vi "Client Console.vi"() -> ()   [LabVIEW 2020]
uses:
  _addons/TCP-Router/_support/tcp-msg type.ctl
  <vilib>/event_ctls.llb/eventvkey.ctl
  <vilib>/Utility/High Resolution Relative Seconds.vi
  <userlib>/_NEVSTOP/Communicable State Machine(CSM)/AdvanceAPI/CSM - Keywords.vi
  <userlib>/_NEVSTOP/Communicable State Machine(CSM)/_Shared/Trim Single-line Text.vi
  <userlib>/_NEVSTOP/Communicable State Machine(CSM)/addons/API-String-Arugments-Support/API String Arguments Support.lvlib
  <userlib>/_NEVSTOP/Communicable State Machine(CSM)/Communicable State Machine.lvlib
  <userlib>/_NEVSTOP/Communicable State Machine(CSM)/addons/INI-Static-Variable-Support/INI-Static-Variable-Support.lvlib
  _addons/TCP-Router/CSM-TCP-Router.lvlib
  <userlib>/_NEVSTOP/Communicable State Machine(CSM)/_Shared/CSM Shared.lvlib
panel:
  out "History Length(Char)":i32
  out "TCP LoopTime(s)":dbl format="%#_3g"
  out "Queue LoopTime(s)":dbl format="%#_3g"
  out "#Queue Backog":i32
  in  "Exit":bool
  out "Console":string
  in  "Command":string caption="$"
  out "To Who":string
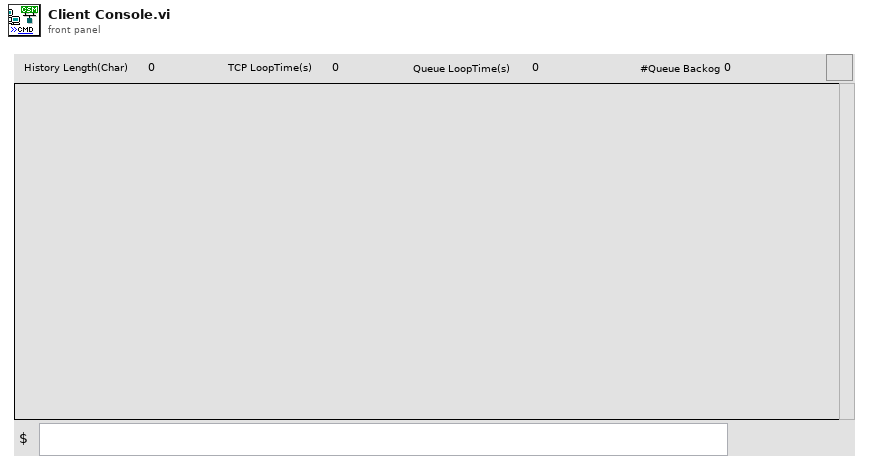
[diagram p1: front panel]
types:
  T1 = typedef "CSM-TCP-Router.lvlib/tcp-msg type.ctl" = enum8{"info", "error", "cmd", "cmd-resp", "resp", "async-resp", "status", "interrupt"}
  T2 = typedef "eventvkey.ctl" = enum16{"ASCII", "Enter", "Return", "Shift", "Ctrl", "Alt", "Cmd", "Opt", "Caps", "NumLock", "Clear", "Break", "Up", "Down", "Left", "Right", "Insert", "Delete", "Home", "End", "PageUp", "PageDown", "Escape", "Help", "Pause", "ScrollLock", "F1", "F2", "F3", "F4", "F5", "F6", "F7", "F8", "F9", "F10", "F11", "F12", "F13", "F14", "F15", "F16", "F17", "F18", "F19", "F20", "F21", "F22", "F23", "F24", "Play", "VolumeUp", "VolumeDown", "Mute", "Two Byte Char"}
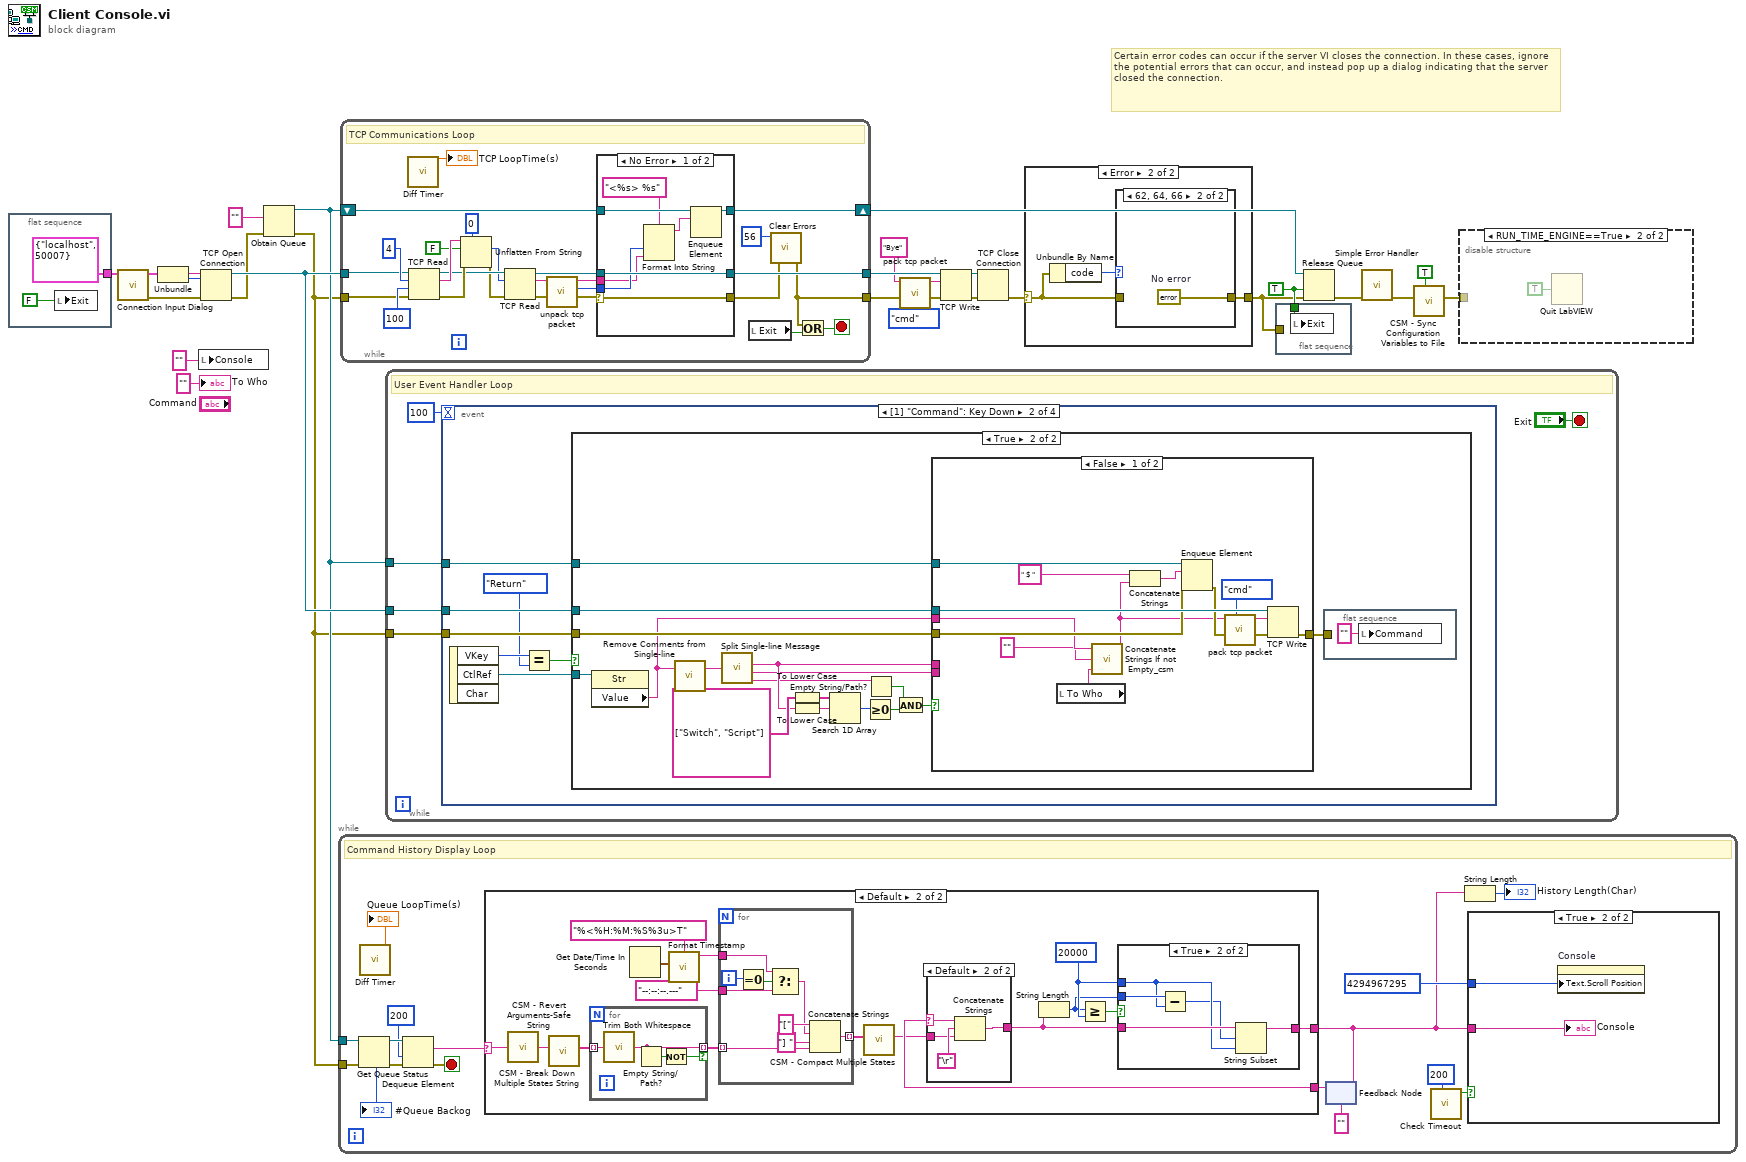
[diagram p0: block diagram]
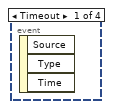
[diagram p7: hidden frame]
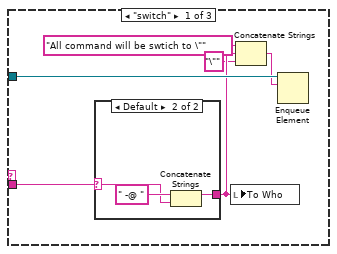
[diagram p10: hidden frame]
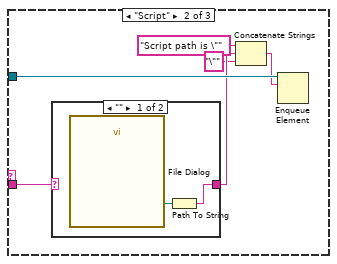
[diagram p12: hidden frame]
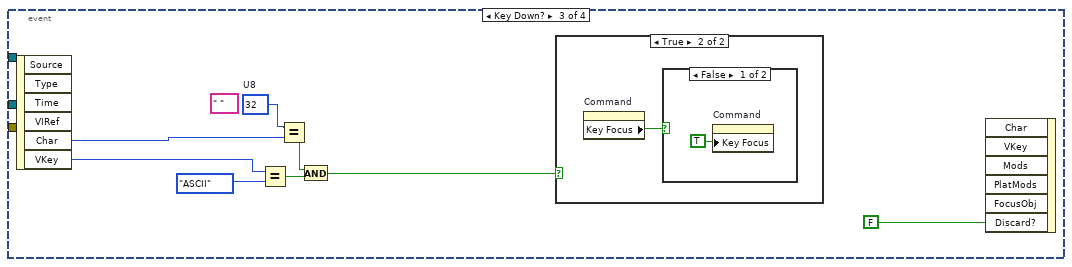
[diagram p14: hidden frame]
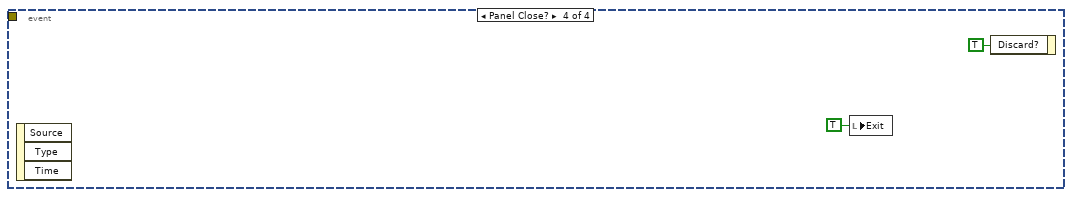
[diagram p17: hidden frame]
diagram:
  w6 = TRUE ("force destroy? (F)")
  # "Certain error codes can occur if the server VI closes the connection. In these cases, ignore the potential errors that can occur, and instead pop up a dialog indicating that the server closed the connection."
  n1 = flat-sequence {
    tunnel: [cluster{"IP Address":string, "Port":u16} {"IP Address"="localhost", "Port"=50007} ("Connection Info")] -> w16
    frame #0 {
      n2 = local write "Exit"(FALSE ("exit")) -> ()
    }
  }
  n3 = call "Connection Input Dialog.vi"("Connection Info"=w16) -> ("Error out"=w15:errorcluster, "Connection Info output"=w14:cluster{"IP Address":string, "Port":u16})  [unwired: 9 in]
  n4 = Unbundle(w14) -> ("IP Address"=w13:string, "Port"=w12:u16)
  n5 = local write "Console"("" ("data out")) -> ()
  n6 = TCP Open Connection(address=w13, remote port or service name=w12, error in (no error)=w15) -> (connection ID=w21:refnum<k5>, error out=w9:errorcluster)  [unwired: 2 in]
  n7 = Obtain Queue(element data type="" ("name (unnamed)"), error in (no error)=w9) -> (queue out=w19:refnum<queue>, error out=w8:errorcluster)  [unwired: 3 in, 1 out]
  n8 = while {
    tunnel: w8 -> [w41]
    tunnel: w19 -> [w45]
    stop <- w44 stop-if-true
    # "Command History Display Loop"
    n9 = Get Queue Status(queue=w45, error in (no error)=w41) -> (queue out=w42:refnum<queue>, error out=w40:errorcluster, # elements in queue=→"#Queue Backog":i32)  [unwired: 1 in, 5 out]
    n10 = call "Diff Timer.vi"() -> ("time diff(s)"=→"Queue LoopTime(s)":dbl)  [unwired: 10 in, 1 out]
    n11 = Dequeue Element(queue=w42, timeout in ms (-1)=200, error in (no error)=w40) -> (element=w43:string, error out=w44:errorcluster)  [unwired: 2 out]
    n12 = feedback #1("") -> (w37:string)
    n13 = case shown="Default" w43 {
      selector: w43 -> [_ w53]
      tunnel: w37 -> [w48 w63]
      tunnel: [w48 w64] -> w33
      frame "" {
      }
      frame Default {
        w61 = 20000 ("length 2")
        n14 = call <userlib>:"CSM - Revert Arguments-Safe String.vi"("Safe Argurment String"=w53) -> ("Origin Argurment String"=w55:string)  [unwired: 8 in]
        n15 = call <userlib>:"CSM - Break Down Multiple States String.vi"("States"=w55) -> ("Multiple States"=w54:string[])  [unwired: 10 in]
        n16 = for {
          tunnel: w54 -> [w77] mode=indexing
          tunnel: [w76] -> w52 mode=indexing if=w74
          n17 = call <userlib>:"Trim Both Whitespace.vi"("string"=w77) -> ("trimmed string"=w76:string)  [unwired: 1 in]
          n18 = Empty String/Path?(string/path=w76) -> (empty?=w75:bool)
          n19 = Not(x=w75) -> (.not. x?=w74:bool)
        }
        n20 = Get Date/Time In Seconds() -> (seconds since 1Jan1904=w56:timestamp)
        n21 = call <userlib>:"Format Timestamp.vi"("timestamp"=w56, "format string"="%<%H:%M:%S%3u>T") -> ("String"=w58:string)  [unwired: 9 in]
        n22 = for {
          tunnel: w58 -> [w67]
          tunnel: [w71] -> w51 mode=indexing
          tunnel: w52 -> [w70] mode=indexing
          tunnel: "--:--:--.---" ("format string") -> [w66]
          i -> [w69]
          n23 = Equal To 0?(x=w69) -> (x = 0?=w68:bool)
          n24 = Select(t=w67, s=w68, f=w66) -> (s? t:f=w65:string)
          n25 = Concatenate Strings("[" ("string"), w65, "] " ("string"), w70) -> (w71:string)
        }
        n26 = call <userlib>:"CSM - Compact Multiple States.vi"("Multiple States"=w51) -> ("States"=w50:string)  [unwired: 9 in]
        n27 = case shown="Default" w63 {
          selector: w63 -> [_ w86]
          tunnel: [w84 w87] -> w62
          tunnel: w50 -> [w84 w85]
          frame "" {
          }
          frame Default {
            n28 = Concatenate Strings(w86, "\r", w85) -> (w87:string)
          }
        }
        n29 = String Length(string=w62) -> (length=w59:i32)
        n30 = Greater Or Equal?(x=w59, y=w61) -> (x >= y?=w60:bool)
        n31 = case shown="True" w60 {
          tunnel: [w78 w83] -> w64
          tunnel: w62 -> [w78 w82]
          tunnel: w61 -> [_ w80]
          tunnel: w59 -> [_ w81]
          frame False {
          }
          frame True {
            n32 = Subtract(x=w81, y=w80) -> (x-y=w79:i32)
            n33 = String Subset(string=w82, offset (0)=w79, length (rest)=w80) -> (substring=w83:string)
          }
        }
      }
    }
    n34 = feedback-in #1(w33) -> ()
    n35 = call <userlib>:"Check Timeout.vi"("Timeout Expected(ms)"=200) -> ("Timeout"=w31:bool)  [unwired: 7 in]
    n36 = String Length(string=w33) -> (length=→"History Length(Char)":i32)
    n37 = case shown="True" w31 {
      tunnel: u32 4294967295 ("Text.Scroll Position") -> [_ w47]
      tunnel: w33 -> [_ w46]
      frame False {
      }
      frame True {
        n38 = property on="Console" class="Str"("Text.Scroll Position"=w47) -> ()  [unwired: 2 in, 2 out]
        "Console" <- w46
      }
    }
  }
  n39 = while {
    tunnel: w8 -> [w94]
    tunnel: w21 -> [w95]
    tunnel: [w113] -> w26
    tunnel: [w107] -> w24
    shift-right: [w109] -> w7
    shift-left: w19 -> [w110]
    stop <- w108 stop-if-true
    # "TCP Communications Loop"
    n40 = call "Diff Timer.vi"() -> ("time diff(s)"=→"TCP LoopTime(s)":dbl)  [unwired: 10 in, 1 out]
    n41 = TCP Read(connection ID=w95, bytes to read=4, error in (no error)=w94, 9:100 ("timeout ms (1000)")) -> (connection ID out=w103:refnum<k5>, data out=w104:string, error out=w105:errorcluster)  [unwired: 1 in]
    n42 = Unflatten From String(type=0, binary string=w104, data includes array or string size? (T)=FALSE, error in (no error)=w105) -> (value=w101:i32, error out=w100:errorcluster)  [unwired: 2 out]
    n43 = TCP Read(connection ID=w103, bytes to read=w101, error in (no error)=w100) -> (connection ID out=w92:refnum<k5>, data out=w102:string, error out=w93:errorcluster)  [unwired: 2 in]
    n44 = call "unpack tcp packet.vi"("TCP Pack"=w102) -> ("tcp-message-type"=w90:T1, "String"=w91:string)  [unwired: 9 in]
    n45 = case shown="No Error" w93 {
      selector: w93 -> [w120 w124]
      tunnel: w92 -> [w121 w123]
      tunnel: [w121 w123] -> w113
      tunnel: [w120 w124] -> w112
      tunnel: w91 -> [w116 _]
      tunnel: w110 -> [w119 w122]
      tunnel: [w118 w122] -> w109
      tunnel: w90 -> [w117 _]
      frame No Error {
        n46 = Format Into String(format string="<%s> %s", w117, w116) -> (resulting string=w115:string)  [unwired: 2 in, 1 out]
        n47 = Enqueue Element(queue=w119, element=w115) -> (queue out=w118:refnum<queue>)  [unwired: 2 in, 2 out]
      }
      frame Error {
      }
    }
    n48 = local read "Exit"() -> (w106:bool)
    n49 = call <vilib>:"Clear Errors.vi"("error in (no error)"=w112, "specific error code to clear (0: all)"=56) -> ("error out"=w107:errorcluster)  [unwired: 4 in, 1 out]
    n50 = Or(x=w107, y=w106) -> (x .or. y?=w108:bool)
  }
  n51 = while {
    tunnel: w21 -> [w129]
    tunnel: w8 -> [w128]
    tunnel: w19 -> [w126]
    stop <- "Exit" stop-if-true
    # "User Event Handler Loop"
    n52 = event shown="[1] \"Command\": Key Down" {
      selector: _ -> [_ _ _ _]
      dyn-events: _ -> [_ _ _ _]
      timeout: 100 -> [_ _ _ _]
      tunnel: w129 -> [_ w136 _ _]
      tunnel: w128 -> [_ w134 _ _]
      tunnel: w126 -> [_ w135 _ _]
      event Timeout {
        n53 = event-data() -> ()  [unwired: 1 in, 3 out]
      }
      event "Command": Key Down {
        n54 = event-data() -> ("VKey"=w132:T2, "CtlRef"=w133:refnum<vi>)  [unwired: 1 in, 1 out]
        n55 = Equal?(x=w132, y=eventvkey."Return") -> (x = y?=w130:bool)
        n56 = case shown="True" w130 {
          tunnel: w136 -> [_ w153]
          tunnel: w135 -> [_ w152]
          tunnel: w134 -> [_ w151]
          tunnel: w133 -> [_ w150]
          frame False {
          }
          frame True {
            n57 = property class="Str"(reference=w150) -> ("Value"=w147:string)  [unwired: 1 in, 2 out]
            n58 = call <userlib>:"Remove Comments from Single-line.vi"("single-line text"=w147) -> ("single-line text without comments"=w148:string)  [unwired: 2 in]
            n59 = call <userlib>:"Split Single-line Message.vi"("single-line text"=w148) -> ("state"=w145:string, "args"=w137:string, "source/target"=w138:string)  [unwired: 6 in, 1 out]
            n60 = To Lower Case(string=string[] ["Switch", "Script"] ("hostname")) -> (all lower case string=w140:string[])
            n61 = To Lower Case(string=w145) -> (all lower case string=w139:string)
            n62 = Search 1D Array(1D array=w140, element=w139) -> (index of element=w144:i32)  [unwired: 1 in]
            n63 = Greater Or Equal To 0?(x=w144) -> (x >= 0?=w143:bool)
            n64 = Empty String/Path?(string/path=w138) -> (empty?=w142:bool)
            n65 = And(x=w142, y=w143) -> (x .and. y?=w141:bool)
            n66 = case shown="False" w141 {
              tunnel: w153 -> [w166 _]
              tunnel: w152 -> [w165 w169]
              tunnel: w151 -> [w161 w170]
              tunnel: [w160 w170] -> w149
              tunnel: w147 -> [w159 _]
              tunnel: w145 -> [_ w167]
              tunnel: w137 -> [_ w168]
              frame False {
                n67 = local read "To Who"() -> (w156:string)
                n68 = call <userlib>:"Concatenate Strings If not Empty_csm.vi"("String"=w156, "seperator(:)"="", "prefix"=w159) -> ("result"=w158:string)  [unwired: 2 in]
                n69 = Concatenate Strings(" $ " ("string"), w158) -> (w163:string)
                n70 = Enqueue Element(queue=w165, element=w163, error in (no error)=w161) -> (error out=w162:errorcluster)  [unwired: 1 in, 2 out]
                n71 = call "pack tcp packet.vi"("tcp-message-type"=tcp-msg_type."cmd", "String"=w158) -> ("TCP Pack"=w155:string)  [unwired: 9 in]
                n72 = TCP Write(connection ID=w166, data in=w155, error in (no error)=w162) -> (error out=w160:errorcluster)  [unwired: 1 in, 2 out]
              }
              frame True {
                n73 = case shown="Default" w167 {
                  tunnel: w169 -> [w175 w184 _]
                  tunnel: w168 -> [w176 w185 _]
                  frame "switch" {
                    n74 = case shown="Default" w176 {
                      selector: w176 -> [_ w177]
                      tunnel: [_ w178] -> w174
                      frame "" {
                      }
                      frame Default {
                        n75 = Concatenate Strings(" -@ " ("To Who"), w177) -> (w178:string)
                      }
                    }
                    n76 = local write "To Who"(w174) -> ()
                    n77 = Concatenate Strings("All command will be swtich to \"" ("string"), w174, "\"" ("string")) -> (w173:string)
                    n78 = Enqueue Element(queue=w175, element=w173) -> ()  [unwired: 2 in, 3 out]
                  }
                  frame "Script" {
                    n79 = case shown="\"\"" w185 {
                      selector: w185 -> [_ w188]
                      tunnel: [w186 w188] -> w183
                      frame "" {
                        n80 = call "File Dialog"() -> ("selected path"=w187:path)  [unwired: 12 in, 3 out]
                        n81 = Path To String(path=w187) -> (string=w186:string)
                      }
                      frame Default {
                      }
                    }
                    n82 = Concatenate Strings("Script path is \"" ("string"), w183, "\"" ("string")) -> (w182:string)
                    n83 = Enqueue Element(queue=w184, element=w182) -> ()  [unwired: 2 in, 3 out]
                  }
                  frame Default {
                  }
                }
              }
            }
            n84 = flat-sequence {
              tunnel: w149 -> [_]
              frame #0 {
                n85 = local write "Command"("" ("Command")) -> ()
              }
            }
          }
        }
      }
      event Key Down? {
        (unwired) " "
        w192 = u8 32  # U8
        n86 = event-data() -> ("Char"=w193:i16, "VKey"=w195:T2)  [unwired: 1 in, 4 out]
        n87 = Equal?(x=w195, y=eventvkey."ASCII" ("VKey")) -> (x = y?=w194:bool)
        n88 = Equal?(x=w192, y=w193) -> (x = y?=w191:bool)
        n89 = And(x=w191, y=w194) -> (x .and. y?=w190:bool)
        n90 = case shown="True" w190 {
          frame False {
          }
          frame True {
            n91 = property on="Command" class="Str"() -> ("Key Focus"=w198:bool)  [unwired: 2 in, 2 out]
            n92 = case shown="False" w198 {
              frame False {
                n93 = property on="Command" class="Str"("Key Focus"=TRUE) -> ()  [unwired: 2 in, 2 out]
              }
              frame True {
              }
            }
          }
        }
        n94 = event-data("Discard?"=FALSE) -> ()  [unwired: 6 in, 1 out]
      }
      event Panel Close? {
        n95 = event-data() -> ()  [unwired: 1 in, 3 out]
        n96 = local write "Exit"(TRUE ("exit")) -> ()
        n97 = event-data("Discard?"=TRUE) -> ()  [unwired: 1 in, 1 out]
      }
    }
  }
  n98 = call "pack tcp packet.vi"("tcp-message-type"=tcp-msg_type."cmd", "String"="Bye") -> ("TCP Pack"=w2:string)  [unwired: 9 in]
  n99 = TCP Write(connection ID=w26, data in=w2, error in (no error)=w24) -> (connection ID out=w27:refnum<k5>, error out=w25:errorcluster)  [unwired: 1 in, 1 out]
  n100 = TCP Close Connection(connection ID=w27, error in (no error)=w25) -> (error out=w5:errorcluster)  [unwired: 1 in, 1 out]
  n101 = case shown="Error" w5 {
    selector: w5 -> [w202 w204]
    tunnel: [w202 w203] -> w3
    frame No Error {
    }
    frame Error {
      n102 = Unbundle By Name(w204) -> ("code"=w205:i32)
      n103 = case shown="62, 64, 66" w205 {
        tunnel: w204 -> [w206 _]
        tunnel: [w206 w207] -> w203
        frame Default {
        }
        frame 62, 64, 66 {
          w207 = errorcluster {"status"=FALSE, "code"=0, "source"=""}  # No error
        }
      }
    }
  }
  n104 = flat-sequence {
    tunnel: w6 -> [w208]
    tunnel: w3 -> [_]
    frame #0 {
      n105 = local write "Exit"(w208) -> ()
    }
  }
  n106 = Release Queue(queue=w7, force destroy? (F)=w6, error in (no error)=w3) -> (error out=w4:errorcluster)  [unwired: 2 out]
  n107 = call <vilib>:"Simple Error Handler.vi"("error in (no error)"=w4) -> ("error out"=w17:errorcluster)  [unwired: 4 in, 4 out]
  n108 = call <userlib>:"CSM - Sync Configuration Variables to File.vi"("All Temp Variable to Default Ini(F)"=TRUE, "error in (no error)"=w17) -> ("error out"=w11:errorcluster)  [unwired: 7 in]
  n109 = disable-structure shown="RUN_TIME_ENGINE==True" {
    disable-tunnel: w11 -> [_ _]
    frame condition #0 (active) {
    }
    frame condition #1 {
      n110 = Quit LabVIEW(quit? (T)=TRUE) -> ()
    }
  }
  "To Who" <- "" ("hostname")
